vi "Actual Record Length Core.vi"(8 "error in (no error)":errorcluster, 11 "IVI_Scope in":refnum<class "IVI_Scope.lvclass">) -> (0 "error out":errorcluster, 2 "actual record length":i32 caption="actual record length (samples)", 3 "IVI_Scope out":refnum<class "IVI_Scope.lvclass">)   [LabVIEW 2015, in "IVI_Scope.lvlib" / "IVI_Scope.lvclass"]
doc: "This VI returns the actual number of points the oscilloscope acquires for each channel. After you configure the oscilloscope for an acquisition, call this VI to determine the size of the waveforms that the oscilloscope acquires. The value is greater than or equal to the minimum number of points you specify in the IviScope Configure Acquisition Record VI. \nYou can use this value as the Waveform Size parameter of the IviScope Read Waveform and IviScope Fetch Waveform VIs."
uses:
  IVI_Scope.lvclass
  IVI_Scope.lvclass/IVI_Scope.ctl
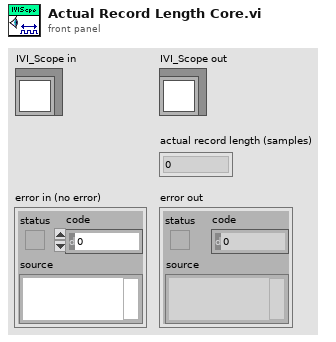
[diagram p1: front panel]
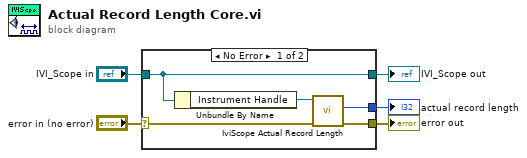
[diagram p0: block diagram]
diagram:
  n1 = case shown="No Error" "error in (no error)" {
    selector: "error in (no error)" -> [w8 w12]
    tunnel: [w7 w12] -> w4
    tunnel: [w10 w11] -> w2
    tunnel: "IVI_Scope in" -> [w10 w11]
    tunnel: [w6 _] -> w1
    frame No Error {
      n2 = Unbundle By Name(w10) -> ("Instrument Handle"=w9:refnum<k15>)
      n3 = call <vilib>:"IviScope Actual Record Length.vi"("error in (no error)"=w8, "instrument handle"=w9) -> ("error out"=w7:errorcluster, "actual record length"=w6:i32)  [unwired: 7 in, 1 out]
    }
    frame Error {
    }
  }
  "error out" <- w4
  "IVI_Scope out" <- w2
  "actual record length" <- w1
